vi "DistributeSelection.vi"(7 "Executed on Frontpanel?":bool, 8 "error in (no error)":errorcluster, 9 "DistributeType":T1(ring), 10 "Panel Ref in":refnum<vi>, 11 "TopLevelDiagram in":refnum<vi>) -> (0 "error out":errorcluster, 2 "Panel Ref out":refnum<vi>, 3 "TopLevelDiagram out":refnum<vi>)   [LabVIEW 2016, in "Align Elements.lvlib"]
doc: "Distribute a selection of elements either on a frontpanel or a block diagram."
uses:
  Align Elements.lvlib
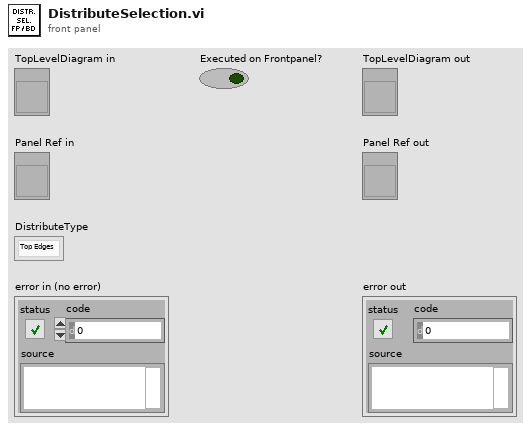
[diagram p1: front panel]
types:
  T1 = enum32{"Top Edges", "Vertical Centers", "Bottom Edges", "Vertical Gap", "Vertical Compress", "Left Edges", "Horizontal Centers", "Right Edges", "Horizontal Gap", "Horizontal Compress"}
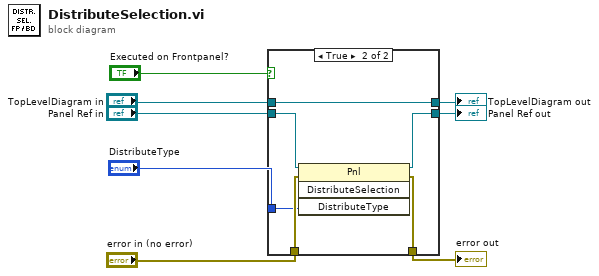
[diagram p0: block diagram]
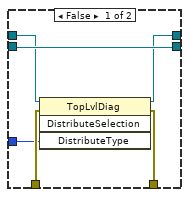
[diagram p2: hidden frame]
diagram:
  n1 = case shown="True" "Executed on Frontpanel?" {
    tunnel: "DistributeType" -> [w9 w15]
    tunnel: "TopLevelDiagram in" -> [w13 w20]
    tunnel: [w12 w20] -> w5
    tunnel: "Panel Ref in" -> [w14 w19]
    tunnel: [w14 w18] -> w6
    tunnel: "error in (no error)" -> [w10 w16]
    tunnel: [w11 w17] -> w7
    frame False {
      n2 = invoke class="TopLvlDiag" method="DistributeSelection"(reference=w13, error in=w10, "DistributeType"=w9) -> (reference out=w12:refnum<vi>, error out=w11:errorcluster)  [unwired: 1 in, 2 out]
    }
    frame True {
      n3 = invoke class="Pnl" method="DistributeSelection"(reference=w19, error in=w16, "DistributeType"=w15) -> (reference out=w18:refnum<vi>, error out=w17:errorcluster)  [unwired: 1 in, 2 out]
    }
  }
  "error out" <- w7
  "Panel Ref out" <- w6
  "TopLevelDiagram out" <- w5
